vi "Draw Rectangle by Roatate Angle.vi"(6 "Draw Para":T1={"fill?(F)"=TRUE, "color(black)"=0, "pen"={"Width"=1, "Style"=enum."Solid"}}, 7 "Angle(Deg)":dbl, 8 "错误输入":errorcluster, 9 "Para":cluster{"dx":i16, "dy":i16}={"dx"=10, "dy"=4}, 10 "Center":T2, 11 "Pic in":picture) -> (0 "错误输出":errorcluster, 3 "Pic out":picture)   [LabVIEW 2012, in "Picture Box Tools.lvlib" / "Basic Shape.lvlib"]
uses:
  Basic Shape.lvlib
  Point Custom Control.ctl
  Draw Para Custom Control.ctl
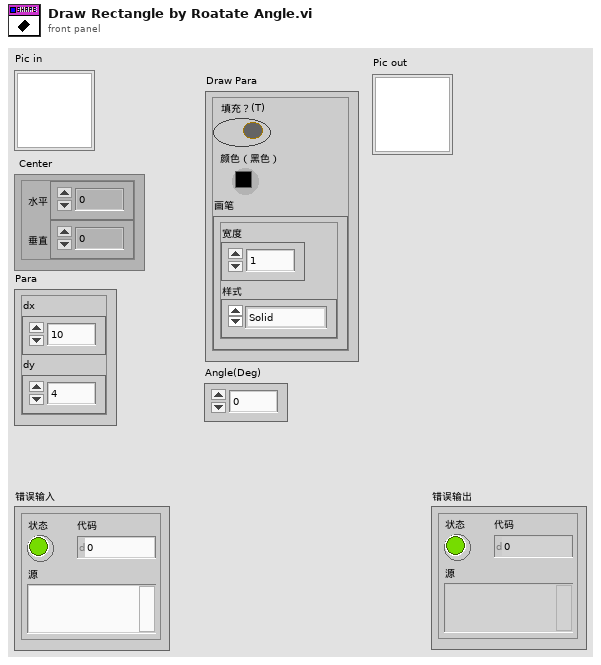
[diagram p1: front panel]
types:
  T1 = typedef "Picture Box Tools.lvlib/Basic Shape.lvlib/Draw Para Custom Control.ctl" = cluster{"fill?(F)":bool, "color(black)":u32, "pen":cluster{"Width":u16, "Style":enum32{"Solid", "Dash", "Dot", "DashDot", "DashDotDot"}}}
  T2 = typedef "Picture Box Tools.lvlib/Basic Shape.lvlib/Point Custom Control.ctl" = cluster{"horizontal":i16, "vertical":i16}
  T3 = cluster{"Width":u16, "Style":enum32{"Solid", "Dash", "Dot", "DashDot", "DashDotDot"}}
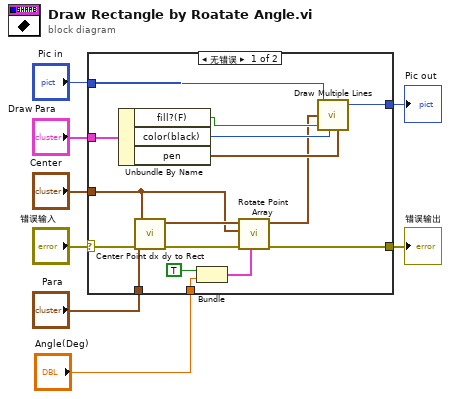
[diagram p0: block diagram]
diagram:
  n1 = case shown="无错误" "错误输入" {
    selector: "错误输入" -> [w24 w26]
    tunnel: [w13 w26] -> w7
    tunnel: "Para" -> [w19 _]
    tunnel: "Center" -> [w15 _]
    tunnel: "Pic in" -> [w18 w25]
    tunnel: [w23 w25] -> w3
    tunnel: "Draw Para" -> [w22 _]
    tunnel: "Angle(Deg)" -> [w10 _]
    frame No Error {
      n2 = Unbundle By Name(w22) -> ("fill?(F)"=w17:bool, "color(black)"=w20:u32, "pen"=w21:T3)
      n3 = call "Center Point dx dy to Rect.vi"("错误输入"=w24, "Para"=w19, "Center"=w15) -> ("错误输出"=w14:errorcluster, "Rect Point Array"=w16:T2[])  [unwired: 7 in]
      n4 = Bundle(TRUE, "Angle(Deg)"=w10) -> (w9:cluster{bool, "Angle(Deg)":dbl})  [unwired: 1 in]
      n5 = call "Rotate Point Array.vi"("Para"=w9, "错误输入"=w14, "Center"=w15, "Point Array"=w16) -> ("错误输出"=w13:errorcluster, "Rotated Absolute Point Array"=w12:T2[])  [unwired: 5 in, 1 out]
      n6 = call <vilib>:"Draw Multiple Lines.vi"("picture"=w18, "line endpoints"=w12, "fill?(F)"=w17, "color(black)"=w20, "pen"=w21) -> ("new picture"=w23:picture)  [unwired: 4 in]
    }
    frame Error {
    }
  }
  "Pic out" <- w3
  "错误输出" <- w7
